vi "Set Result Fied Parameters.vi"(8 "ErrorIn":errorcluster, 11 "VISAIn":refnum<visa-resource-name>) -> (0 "ErrorOut":errorcluster, 3 "VISAOut":refnum<visa-resource-name>)   [LabVIEW 2017]
uses:
  I28 Drivers/I28Drivers.lvlib
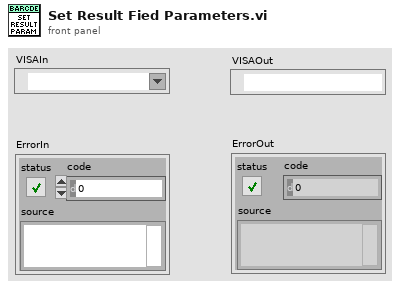
[diagram p1: front panel]
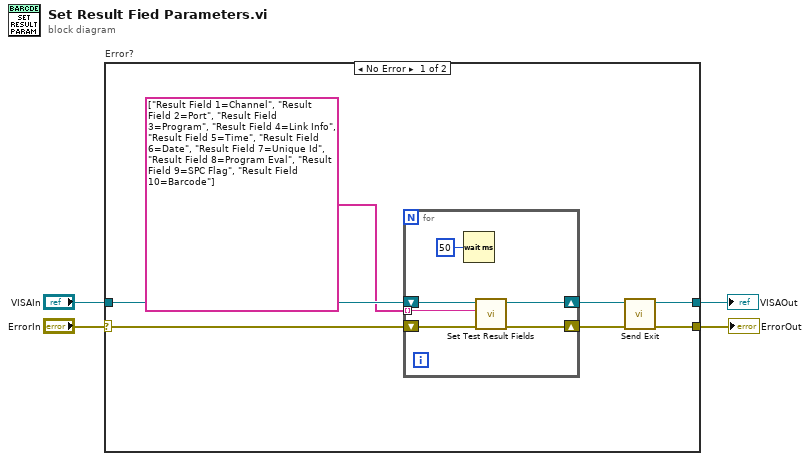
[diagram p0: block diagram]
diagram:
  n1 = case "Error?" shown="No Error" "ErrorIn" {
    selector: "ErrorIn" -> [w10 w18]
    tunnel: "VISAIn" -> [w11 _]
    tunnel: [w6 w18] -> w2
    tunnel: [w5 _] -> w1
    frame No Error {
      n2 = for {
        shift-right: [w12] -> w8
        shift-left: w10 -> [w16]
        tunnel: string[] ["Result Field 1=Channel", "Result Field 2=Port", "Result Field 3=Program", "Result Field 4=Link Info", "Result Field 5=Time", "Result Field 6=Date", "Result Field 7=Unique Id", "Result Field 8=Program Eval", "Result Field 9=SPC Flag", "Result Field 10=Barcode"] -> [w15] mode=indexing
        shift-right: [w13] -> w7
        shift-left: w11 -> [w17]
        n3 = Wait (ms)(milliseconds to wait=u32 50) -> ()  [unwired: 1 out]
        n4 = call "Set Test Result Fields.vi"("ErrorIn"=w16, "Command"=w15, "VISAIn"=w17) -> ("ErrorOut"=w12:errorcluster, "VISAOut"=w13:refnum<visa-resource-name>)  [unwired: 6 in, 1 out]
      }
      n5 = call "Send Exit.vi"("ErrorIn"=w8, "VISAIn"=w7) -> ("ErrorOut"=w6:errorcluster, "VISAOut"=w5:refnum<visa-resource-name>)  [unwired: 7 in, 1 out]
    }
    frame Error {
    }
  }
  "ErrorOut" <- w2
  "VISAOut" <- w1
